vi "vipm_InstallPackages.vi"(8 "error in (no error)":errorcluster, 11 "CommandLine":path[](array[path])=[path ""]) -> (0 "error out":errorcluster, 2 "test details":string, 3 "output to action":string)   [LabVIEW 2017, in "_Try Beta Version of CSMF.lvlib"]
uses:
  c27215ec-4270-4bd3-95c1-6003894111c7.vi
  c27215ec-4270-4bd3-95c1-6003894111c7.vi/4443fd46-6fa0-42fe-b173-791422f8c268.vi
  c27215ec-4270-4bd3-95c1-6003894111c7.vi/6d53486d-9fa3-4d68-a12f-868746fe63e7.vi
  c27215ec-4270-4bd3-95c1-6003894111c7.vi/0f454a58-6c15-4936-bc29-faa145c60f00.vi
  c27215ec-4270-4bd3-95c1-6003894111c7.vi/f527980d-0bc5-43c6-aa3b-2feb9b9409a6.vi
  _Try Beta Version of CSMF.lvlib
  <vilib>/JKI/VIPM API/VIPM API_vipm_api.lvlib
panel:
  # "lava_lib_json_api-1.5.5.41"
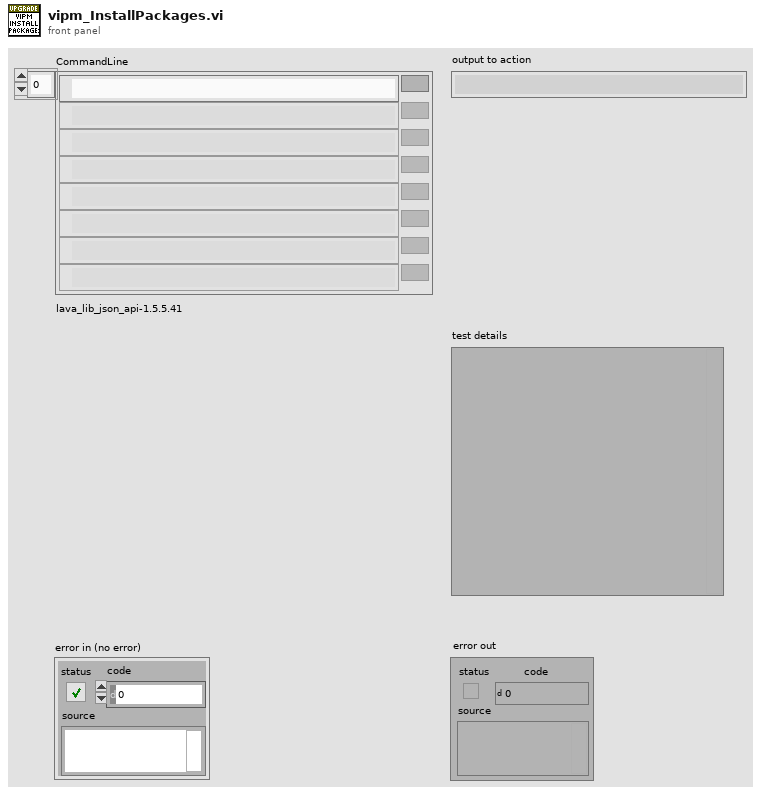
[diagram p1: front panel]
types:
  T1 = typedef "VIPM API_vipm_api.lvlib/Library Contents Cluster_vipm_api.ctl" = cluster{"Package Name":string, "Version":string, "Display Name":string, "Repository Name":string, "Company Name":string, "License Type":string, "Installed":bool, "Deprecated":bool, "Dependency or Conflict Problem":bool, "Downloaded":bool}
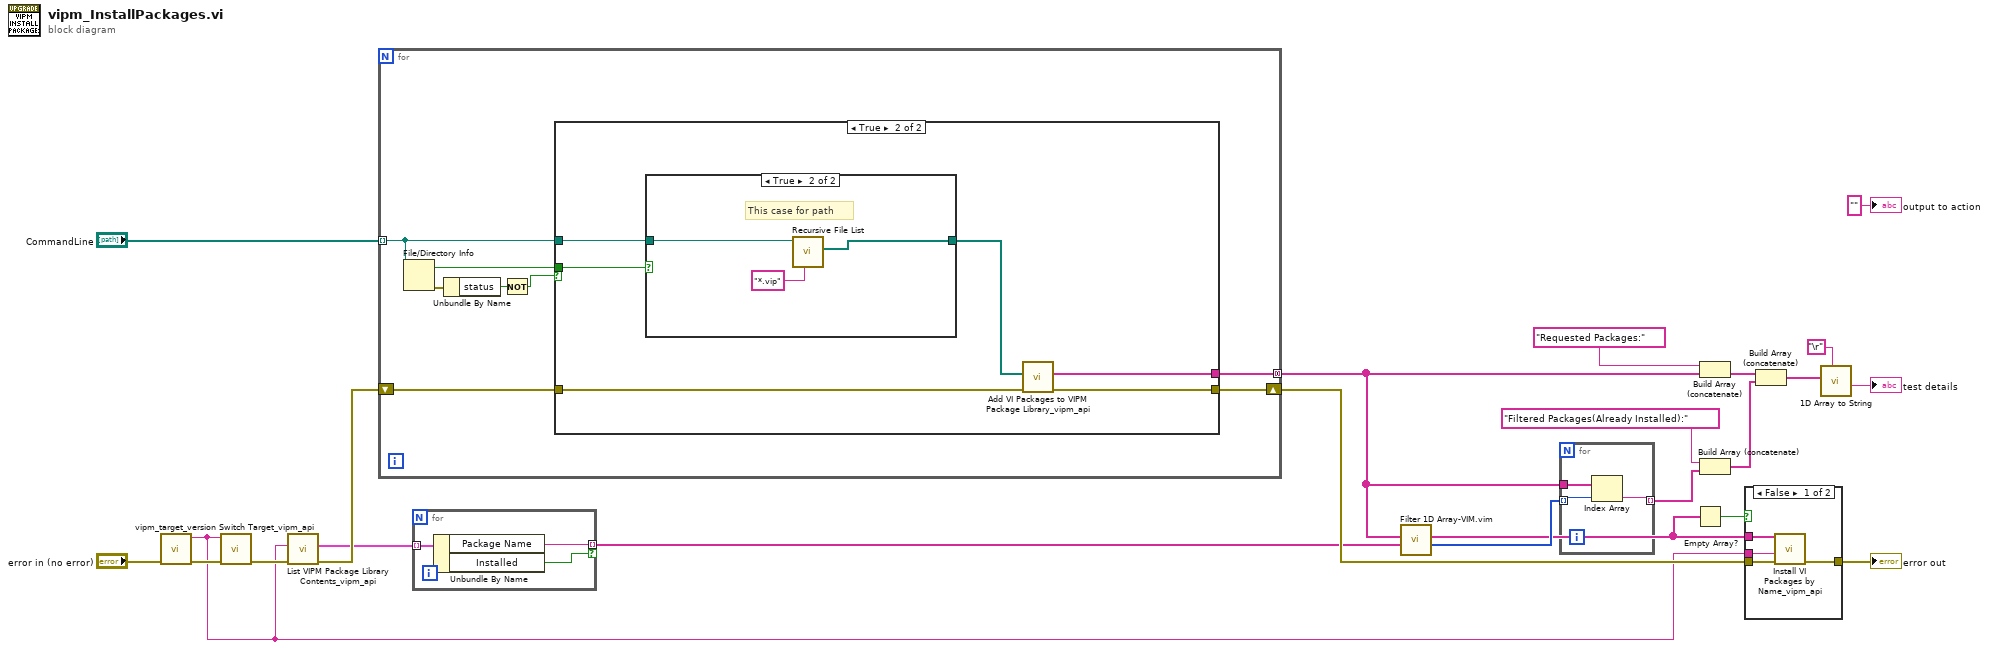
[diagram p0: block diagram]
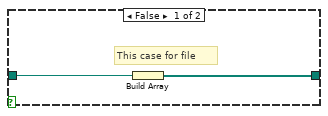
[diagram p4: hidden frame]
diagram:
  n1 = call "vipm_target_version.vi"() -> ("vipm Taget version"=w13:string)  [unwired: 11 in]
  n2 = call <vilib>:"Switch Target_vipm_api.vi"("error in (no error)"="error in (no error)", "LabVIEW Version"=w13) -> ("error out"=w15:errorcluster)  [unwired: 9 in]
  n3 = call <vilib>:"List VIPM Package Library Contents_vipm_api.vi"("error in (no error)"=w15, "LabVIEW Version"=w13) -> ("error out"=w14:errorcluster, "Library Contents []"=w12:T1[])  [unwired: 7 in, 1 out]
  n4 = for {
    tunnel: "CommandLine" -> [w27] mode=indexing
    tunnel: [w29] -> w2 mode=concatenating
    shift-right: [w28] -> w16
    shift-left: w14 -> [w30]
    n5 = File/Directory Info(path=w27) -> (directory=w25:bool, error out=w23:errorcluster)  [unwired: 1 in, 5 out]
    n6 = Unbundle By Name(w23) -> ("status"=w24:bool)
    n7 = Not(x=w24) -> (.not. x?=w26:bool)
    n8 = case shown="True" w26 {
      tunnel: w30 -> [w31 w37]
      tunnel: [_ w36] -> w29
      tunnel: [w31 w35] -> w28
      tunnel: w27 -> [_ w33]
      tunnel: w25 -> [_ w32]
      frame False {
        # "path not exist"
      }
      frame True {
        n9 = case shown="True" w32 {
          tunnel: [w39 w40] -> w34
          tunnel: w33 -> [w38 w42]
          frame False {
            # "This case for file"
            n10 = Build Array(w38) -> (w39:path[])
          }
          frame True {
            # "This case for path"
            n11 = call <vilib>:"Recursive File List.vi"("pattern"="*.vip", "Folder Path"=w42) -> ("All Files in Dir"=w40:path[])  [unwired: 5 in, 4 out]
          }
        }
        n12 = call <vilib>:"Add VI Packages to VIPM Package Library_vipm_api.vi"("error in (no error)"=w37, "Packages to add to VIPM Library (vipc,vip,ogp)"=w34) -> ("error out"=w35:errorcluster, "Package Names Added"=w36:string[])  [unwired: 8 in]
      }
    }
  }
  n13 = for {
    tunnel: w12 -> [w45] mode=indexing
    tunnel: [w44] -> w1 mode=indexing if=w43
    n14 = Unbundle By Name(w45) -> ("Package Name"=w44:string, "Installed"=w43:bool)
  }
  n15 = call "Filter 1D Array-VIM.vim"("Item(s) to Filter"=w1, "Array"=w2) -> ("Filtered Item Indices"=w11:i32[], "Filtered Array"=w4:string[])  [unwired: 5 in]
  n16 = for {
    tunnel: w11 -> [w47] mode=indexing
    tunnel: [w46] -> w8 mode=indexing
    tunnel: w2 -> [w48]
    n17 = Index Array(array=w48, index=w47) -> (element=w46:string)
  }
  n18 = Empty Array?(array=w4) -> (empty?=w3:bool)
  n19 = Build Array (concatenate)("Requested Packages:" ("output to action"), w2) -> (w10:string[])
  n20 = Build Array (concatenate)("Filtered Packages(Already Installed):" ("output to action"), w8) -> (w5:string[])
  n21 = case shown="False" w3 {
    tunnel: [w52 w53] -> w22
    tunnel: w16 -> [w51 w53]
    tunnel: w13 -> [w50 _]
    tunnel: w4 -> [w49 _]
    frame False {
      n22 = call <vilib>:"Install VI Packages by Name_vipm_api.vi"("error in (no error)"=w51, "LabVIEW Version"=w50, "Package Names to Install []"=w49) -> ("error out"=w52:errorcluster)  [unwired: 8 in]
    }
    frame True {
    }
  }
  "error out" <- w22
  n23 = Build Array (concatenate)(w10, w5) -> (w6:string[])
  n24 = call "1D Array to String.vi"("delimiter (Tab)"="\r" ("Carriage Return Constant"), "Array of Strings"=w6) -> ("delimited string"=→"test details":string)  [unwired: 9 in]
  "output to action" <- "" ("output to action")
